vi "Append Numeric Table to Report.vi"(0 "report in":T1, 1 "column width (1)":dbl=1.0 format="%.2f", 2 "measurement system":u16(ring)=2 caption="measurement system for column width (Default)" items=["US", "Metric", "Default"], 5 "column headers":string[](array[string]), 7 "row headers":string[](array[string]), 9 "numerical data":dbl[][](array[numeric]) format="%.2f", 11 "error in (no error)":errorcluster, 12 "format string (%.2f)":string="%.2f", 13 "separate page?":bool, 14 "show grid lines":bool) -> (4 "report out":T1, 15 "error out":errorcluster)   [LabVIEW 2020]
doc: "Appends a 2D array to a report as a table with the given column width. The data type you wire to the <B>text data</B> input determines the polymorphic instance to use."
uses:
  <vilib>/Utility/NIReport.llb/Generate Report Object Reference.ctl
  <vilib>/Utility/NIReport.llb/NI_report.lvclass
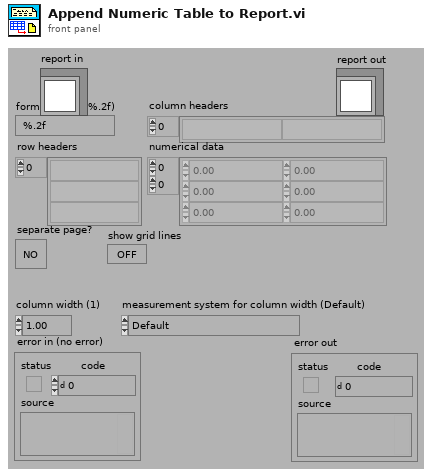
[diagram p1: front panel]
types:
  T1 = typedef "Generate Report Object Reference.ctl" = refnum<class "NI_report.lvclass">
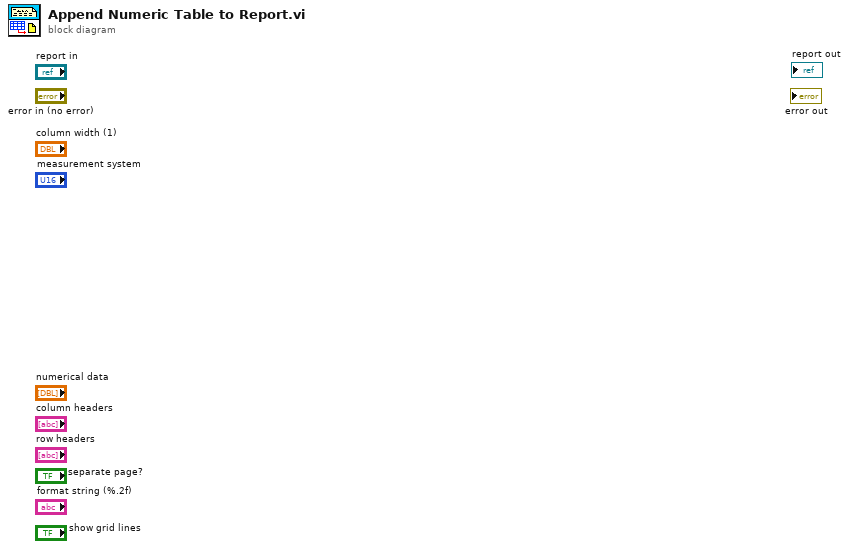
[diagram p0: block diagram]
diagram:
